vi "Send Response.vi"(8 "error in":errorcluster, 9 "Response":variant, 11 "Module in":refnum<class "Module.lvclass">) -> (0 "error out":errorcluster, 3 "Module out":refnum<class "Module.lvclass">)   [LabVIEW 2020, in "Module.lvclass"]
uses:
  Module.lvclass
  Module.lvclass/Module.ctl
  controls/Module response.ctl
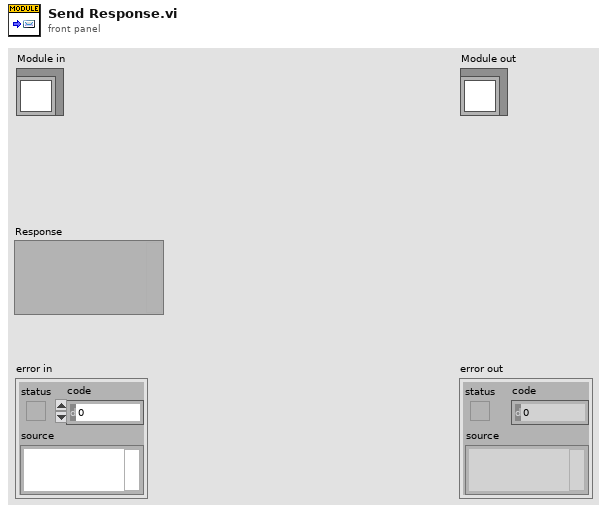
[diagram p1: front panel]
types:
  T1 = typedef "Module response.ctl" = cluster{"ID":string, "Response":variant}
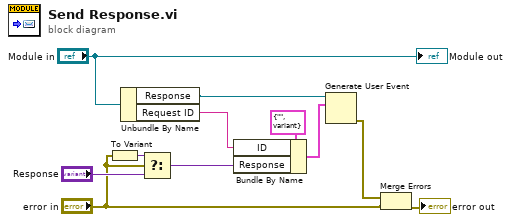
[diagram p0: block diagram]
diagram:
  n1 = To Variant(anything="error in") -> (Variant=w8:variant)
  n2 = Unbundle By Name("Module in") -> ("Response"=w7:refnum<user-event>, "Request ID"=w1:string)
  n3 = Select(t=w8, s="error in", f="Response") -> (s? t:f=w10:variant)
  n4 = Bundle By Name(cluster=T1 {"ID"="", "Response"=variant} ("Module response"), "ID"=w1, "Response"=w10) -> (w6:T1)
  n5 = Generate User Event(user event=w7, event data cluster=w6) -> (error out=w2:errorcluster)  [unwired: 2 in, 1 out]
  n6 = Merge Errors(w2, "error in") -> (→"error out":errorcluster)
  "Module out" <- "Module in"
